vi "Ramp_Lauda_v2.vi"(0 "manual":i32, 1 "Tr_Tj":i32=1, 2 "update":i32, 5 "Tr":dbl[](array[numeric]), 6 "time_manual":dbl, 7 "T_manual":dbl=20.0, 8 "enable":i32, 9 "time_set":dbl[](array[numeric]), 16 "reset":i32, 17 "time_wait":dbl[](array[numeric]), 20 "port":i32=1, 21 "T_sp":dbl[](array[numeric])) -> (4 "elapsed":dbl, 10 "LED_1":bool, 11 "LED_manual":bool, 12 "LED_2":bool, 13 "T0_":dbl, 14 "step":dbl, 15 "LED_stop":bool, 18 "LED_3":bool, 24 "setpoint":dbl, 25 "Tr_out":dbl, 27 "T int":dbl)   [LabVIEW 2016]
uses:
  BERTTA.dll
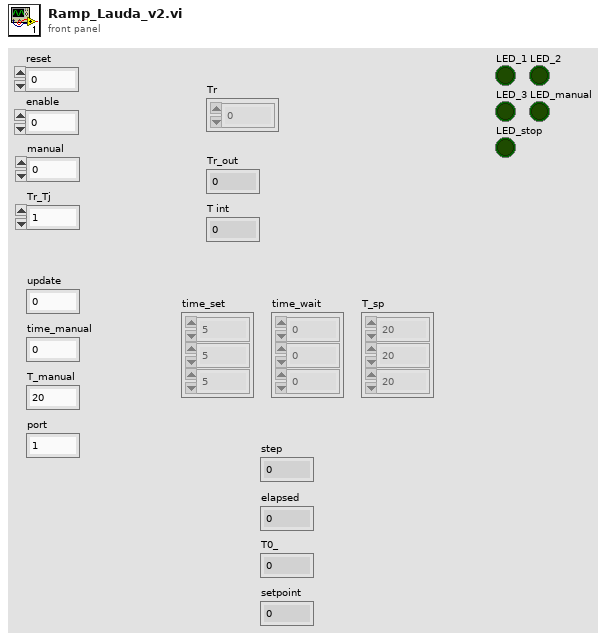
[diagram p1: front panel]
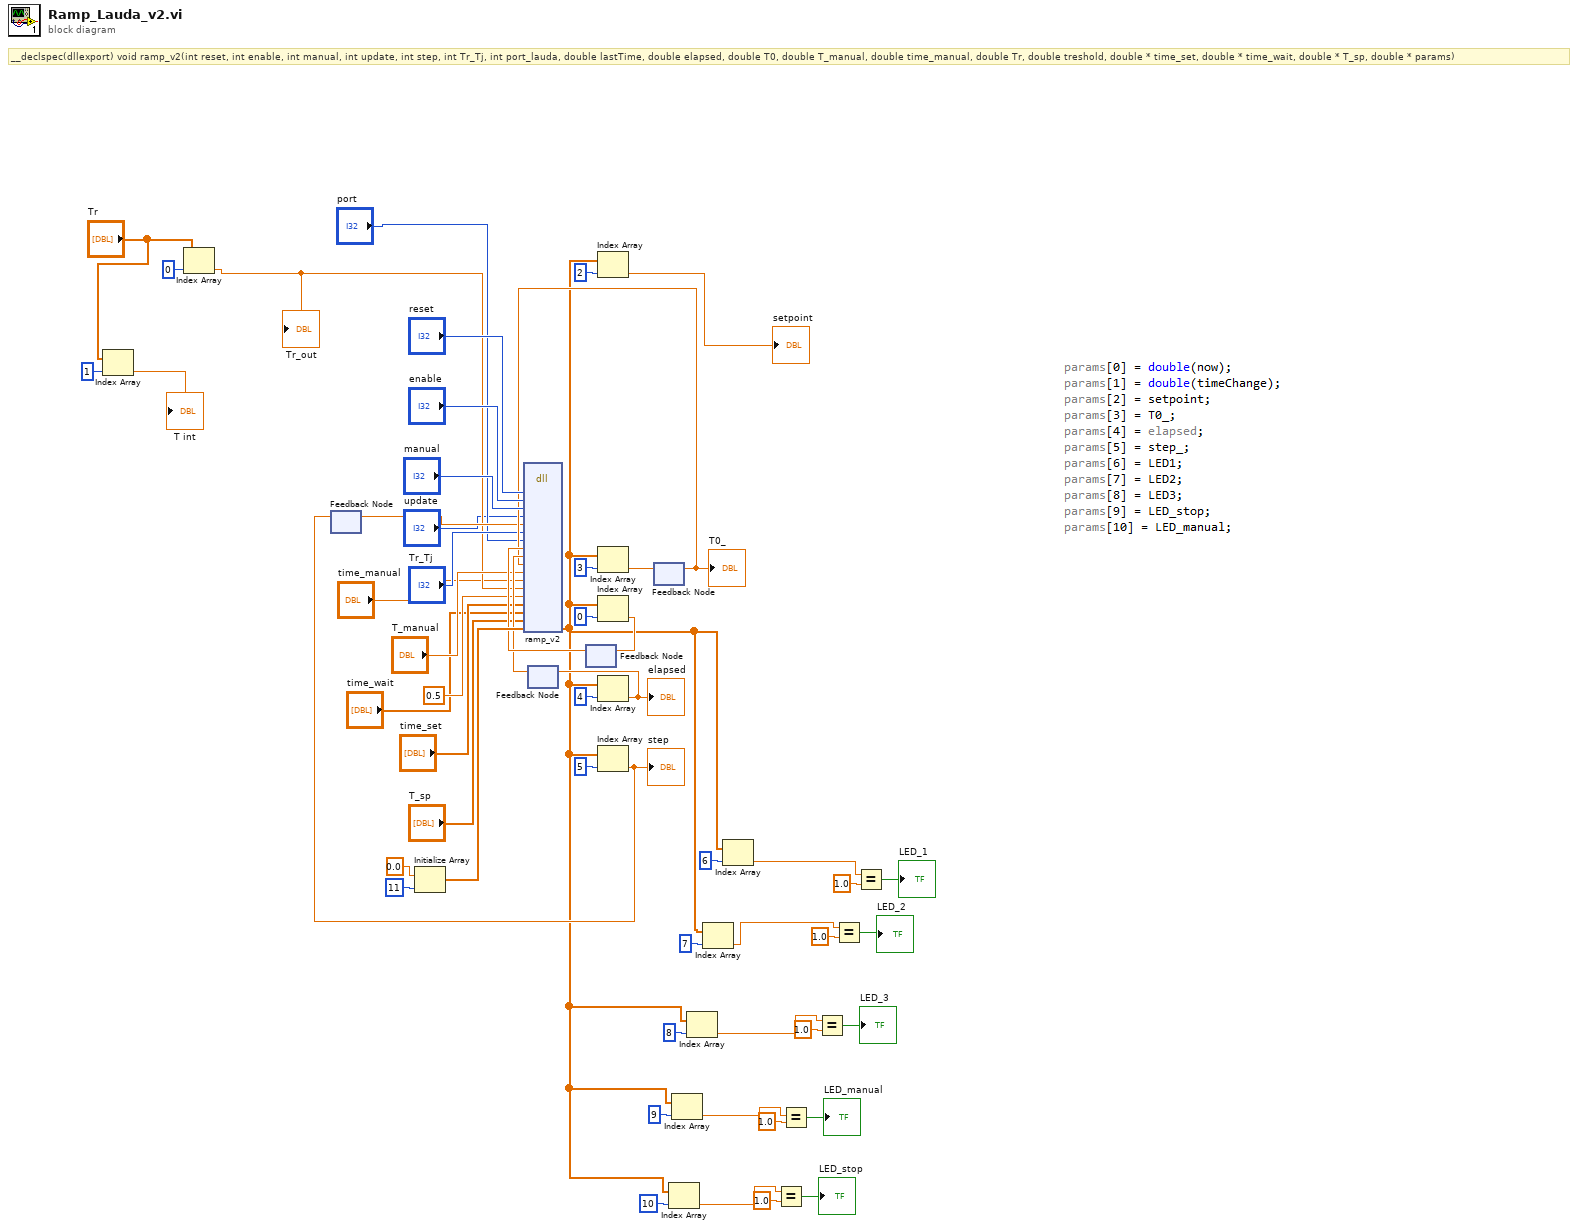
[diagram p0: block diagram]
diagram:
  # "__declspec(dllexport) void ramp_v2(int reset, int enable, int manual, int update, int step, int Tr_Tj, int port_lauda, double lastTime, double elapsed, double T0, double T_manual, double time_manual, double Tr, double treshold, double * time_set, double * time_wait, double * T_sp, double * params)"
  n1 = Index Array(array="Tr", index=1) -> (element=→"T int":dbl)
  n2 = Index Array(array="Tr", index=0) -> (element=w27:dbl)
  "Tr_out" <- w27
  n3 = feedback #1() -> (w35:dbl)  [unwired: 1 in]
  n4 = Initialize Array(0.0 ("element"), 11 ("dimension size")) -> (w50:dbl[])
  n5 = feedback #2() -> (w44:dbl)  [unwired: 1 in]
  n6 = feedback #3() -> (w47:dbl)  [unwired: 1 in]
  n7 = feedback #4() -> (w41:dbl)  [unwired: 1 in]
  "T0_" <- w41
  n8 = dll-call lib="C:/Users/shresplab/OneDrive - Kemira Oyj/Documents/GitHub/Bertta/BERTTA/x64/Debug/BERTTA.dll" fn="ramp_v2"("reset"="reset", "enable"="enable", "manual"="manual", "update"="update", "step"=w35, "Tr_Tj"="Tr_Tj", "port_lauda"="port", "lastTime"=w47, "elapsed"=w44, "T0"=w41, "T_manual"="T_manual", "time_manual"="time_manual", "Tr"=w27, "treshold"=0.5, "time_set"="time_set", "time_wait"="time_wait", "T_sp"="T_sp", "params"=w50) -> ("params"=w18:dbl[])  [unwired: 21 in, 2 out]
  n9 = Index Array(array=w18, index=2) -> (element=→"setpoint":dbl)
  n10 = Index Array(array=w18, index=3) -> (element=w42:dbl)
  n11 = Index Array(array=w18, index=0) -> (element=w48:dbl)
  n12 = feedback-in #3(w48) -> ()
  n13 = Index Array(array=w18, index=4) -> (element=w45:dbl)
  "elapsed" <- w45
  n14 = feedback-in #2(w45) -> ()
  n15 = Index Array(array=w18, index=5) -> (element=w36:dbl)
  "step" <- w36
  n16 = feedback-in #1(w36) -> ()
  n17 = feedback-in #4(w42) -> ()
  n18 = Index Array(array=w18, index=10) -> (element=w8:dbl)
  n19 = Index Array(array=w18, index=9) -> (element=w9:dbl)
  n20 = Index Array(array=w18, index=8) -> (element=w10:dbl)
  n21 = Index Array(array=w18, index=7) -> (element=w11:dbl)
  n22 = Index Array(array=w18, index=6) -> (element=w16:dbl)
  n23 = Equal?(x=w8, y=1.0) -> (x = y?=→"LED_stop":bool)
  n24 = Equal?(x=w9, y=1.0) -> (x = y?=→"LED_manual":bool)
  n25 = Equal?(x=w10, y=1.0) -> (x = y?=→"LED_3":bool)
  n26 = Equal?(x=w11, y=1.0) -> (x = y?=→"LED_2":bool)
  n27 = Equal?(x=w16, y=1.0) -> (x = y?=→"LED_1":bool)
